vi "计算二阶三阶正图像.vi"(1 "正图像筛选门限":dbl, 2 "差分计算一维矩阵":dbl[](array[numeric]), 3 "散斑二维数组行数":i32, 4 "散斑二维数组":dbl[][](array[numeric])) -> (0 "未归一化二阶正图像":dbl[][](array[numeric]))   [LabVIEW 2018]
panel:
  out "未归一化三阶正图像":dbl[][](array[numeric])
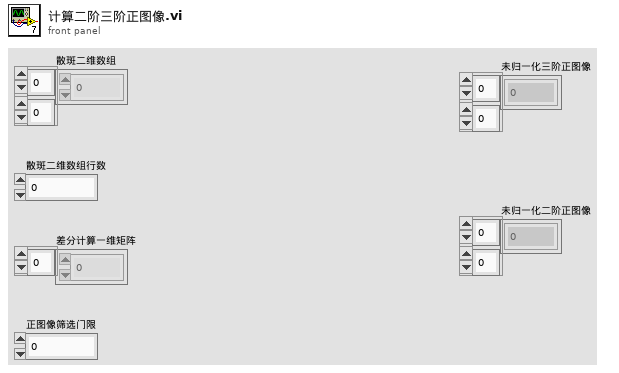
[diagram p1: front panel]
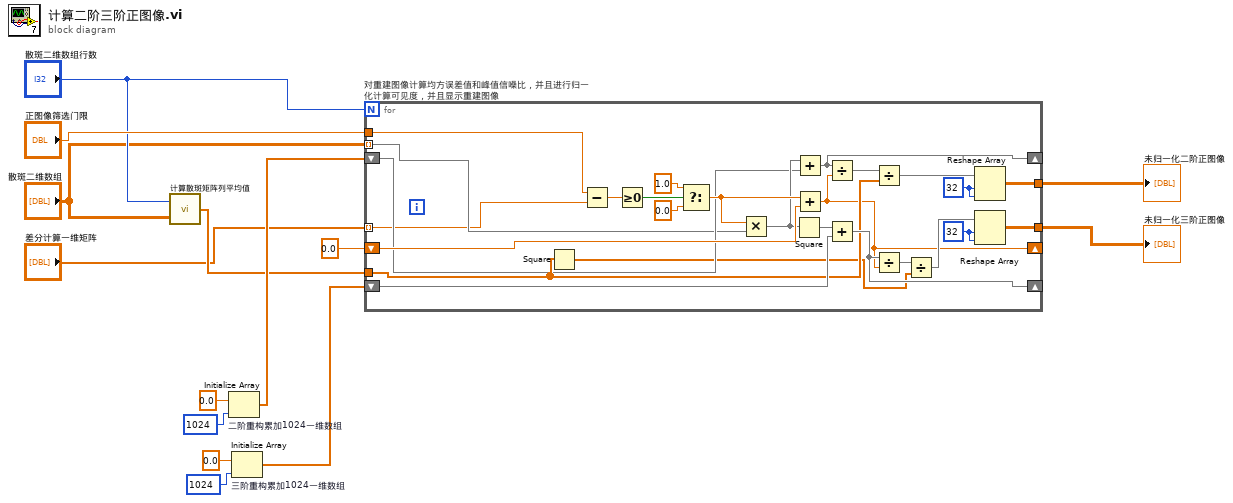
[diagram p0: block diagram]
diagram:
  n1 = call "计算散斑矩阵列平均值.vi"("散斑二维数组"="散斑二维数组", "散斑二维数组行数"="散斑二维数组行数") -> ("散斑二维数组列平均值"=w2:dbl[])
  n2 = Initialize Array "二阶重构累加1024一维数组"(0.0 ("元素"), 1024 ("维数大小")) -> (w7:dbl[])
  n3 = Initialize Array "三阶重构累加1024一维数组"(0.0 ("元素"), 1024 ("维数大小")) -> (w8:dbl[])
  n4 = for "对重建图像计算均方误差值和峰值信噪比，并且进行归一化计算可见度，并且显示重建图像" {
    N: "散斑二维数组行数" -> [_]
    tunnel: "散斑二维数组" -> [w16] mode=indexing
    shift-right: [w22] -> _
    shift-left: w7 -> [w21]
    shift-right: [w18] -> _
    shift-left: 0.0 ("数值") -> [w34]
    tunnel: "正图像筛选门限" -> [w40]
    tunnel: w2 -> [w23]
    shift-right: [w26] -> _
    shift-left: w8 -> [w27]
    tunnel: [w17] -> w5
    tunnel: [w19] -> w6
    tunnel: "差分计算一维矩阵" -> [w15] mode=indexing
    w30 = 32 ("维数大小")
    w33 = 32 ("维数大小")
    n5 = Square(x=w23) -> (x^2=w20:dbl[])
    n6 = Subtract(x=w40, y=w15) -> (x-y=w36:dbl)
    n7 = Greater Or Equal To 0?(x=w36) -> (x >= 0?=w39:bool)
    n8 = Select(t=1.0, s=w39, f=0.0) -> (s? t:f=w35:dbl)
    n9 = Multiply(x=w35, y=w16) -> (x*y=w29:dbl[])
    n10 = Square(x=w29) -> (x^2=w28:dbl[])
    n11 = Add(x=w29, y=w21) -> (x+y=w22:dbl[])
    n12 = Add(x=w35, y=w34) -> (x+y=w18:dbl)
    n13 = Divide(x=w22, y=w18) -> (x/y=w32:dbl[])
    n14 = Add(x=w28, y=w27) -> (x+y=w26:dbl[])
    n15 = Divide(x=w32, y=w23) -> (x/y=w31:dbl[])
    n16 = Divide(x=w26, y=w18) -> (x/y=w25:dbl[])
    n17 = Divide(x=w25, y=w20) -> (x/y=w24:dbl[])
    n18 = Reshape Array(w31, w33, w33) -> (w17:dbl[][])
    n19 = Reshape Array(w24, w30, w30) -> (w19:dbl[][])
  }
  "未归一化三阶正图像" <- w6
  "未归一化二阶正图像" <- w5
